vi "Head.vi"(11 "Boolean IN":bool) -> (3 "Boolean OUT":bool)   [LabVIEW 2025]
panel:
  # "fifnosdfinsdfoin"
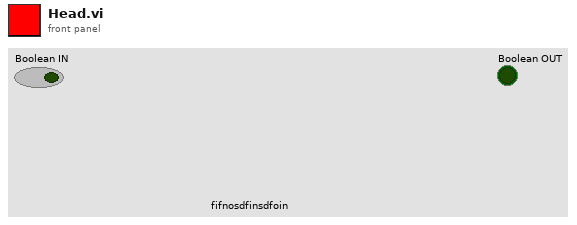
[diagram p1: front panel]
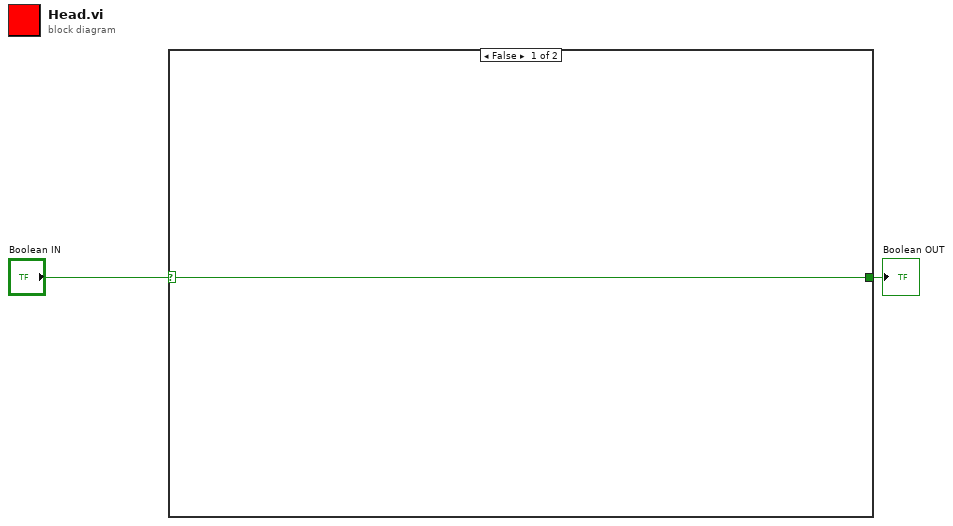
[diagram p0: block diagram]
diagram:
  n1 = case shown="False" "Boolean IN" {
    selector: "Boolean IN" -> [w3 w4]
    tunnel: [w3 w4] -> w1
    frame False {
    }
    frame True {
    }
  }
  "Boolean OUT" <- w1
